vi "Create Settings File.vi"(8 "error in":errorcluster) -> (0 "error out":errorcluster, 3 "named_positions":T1[](array[typedef]))   [LabVIEW 2020, in "Manipulator.lvlib"]
uses:
  Manipulator.lvlib
  Named Position.ctl
panel:
  out "JSON string":string
  out "path":path
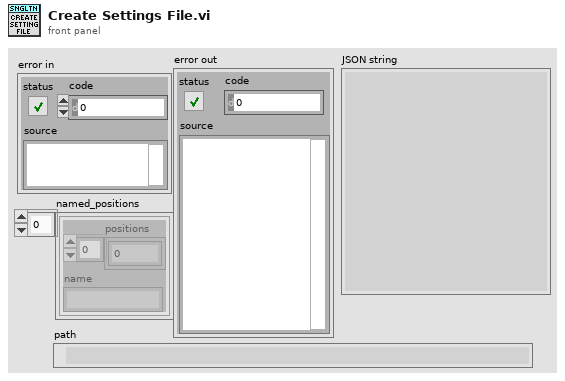
[diagram p1: front panel]
types:
  T1 = typedef "Manipulator.lvlib/Named Position.ctl" = cluster{"positions":dbl[], "name":string}
  T2 = enum16{"open", "replace", "create", "open or create", "replace or create", "replace or create with confirmation"}
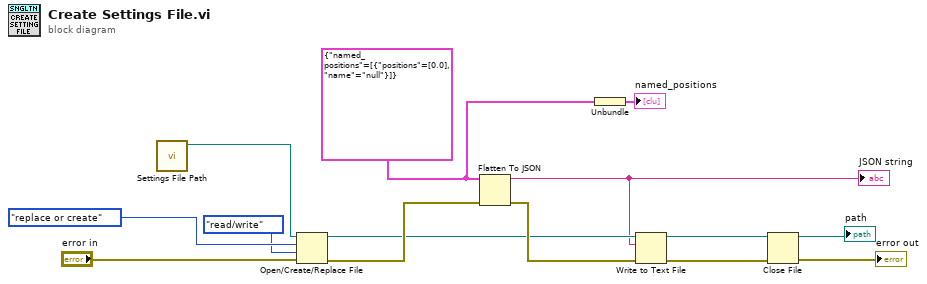
[diagram p0: block diagram]
diagram:
  w2 = cluster{"named_positions":T1[]} {"named_positions"=[{"positions"=[0.0], "name"="null"}]}
  n1 = call "Settings File Path.vi"() -> ("settings path"=w12:path)  [unwired: 11 in]
  n2 = Open/Create/Replace File(file path (use dialog)=w12, error in="error in", operation (0:open)=T2."replace or create", access (0:read/write)=enum16{"read/write", "read-only", "write-only"}."read/write") -> (refnum out=w5:refnum<file>, error out=w8:errorcluster)  [unwired: 2 in, 1 out]
  n3 = Flatten To JSON(anything=w2, error in (no error)=w8) -> (JSON string=w3:string, 11:w7:errorcluster)  [unwired: 1 in]
  "JSON string" <- w3
  n4 = Unbundle(w2) -> ("named_positions"=→"named_positions":T1[])
  n5 = Write to Text File(file (use dialog)=w5, text=w3, error in=w7) -> (refnum out=w4:refnum<file>, error out=w6:errorcluster)  [unwired: 1 in, 1 out]
  n6 = Close File(refnum=w4, error in=w6) -> (path=→"path":path, error out=→"error out":errorcluster)
